vi "lab5_task3_2.vi"() -> ()   [LabVIEW 2021]
uses:
  <vilib>/express/express analysis/Spectral/Block/exnSpectralBlock spectral measurements PSD poly.vi
  <vilib>/express/express analysis/Spectral/Block/exnSpectralBlock spectral measurements PSD DDT.vi
  <vilib>/express/express analysis/Spectral/XNode/ExpressSpectralMeasurementsBlockNode.xnode
  <vilib>/Analysis/NI_AALPro.lvlib
panel:
  out "mass(g)":dbl
  out "number samples":dbl
  in  "Duration(s)":dbl=10000.0
  in  "Sampling rate(hz)":dbl=10000.0
  in  "stop":bool
  out "Intensity Chart":dbl[][](graph)
  out "Power spectral density":dynamicdata(graph)
  in  "# bins":i32
  out "Histogram Graph":T1(graph)
  out "rms":dbl
  out "peak to peak":dbl
  out "mean":dbl
  out "data":dynamicdata(graph)
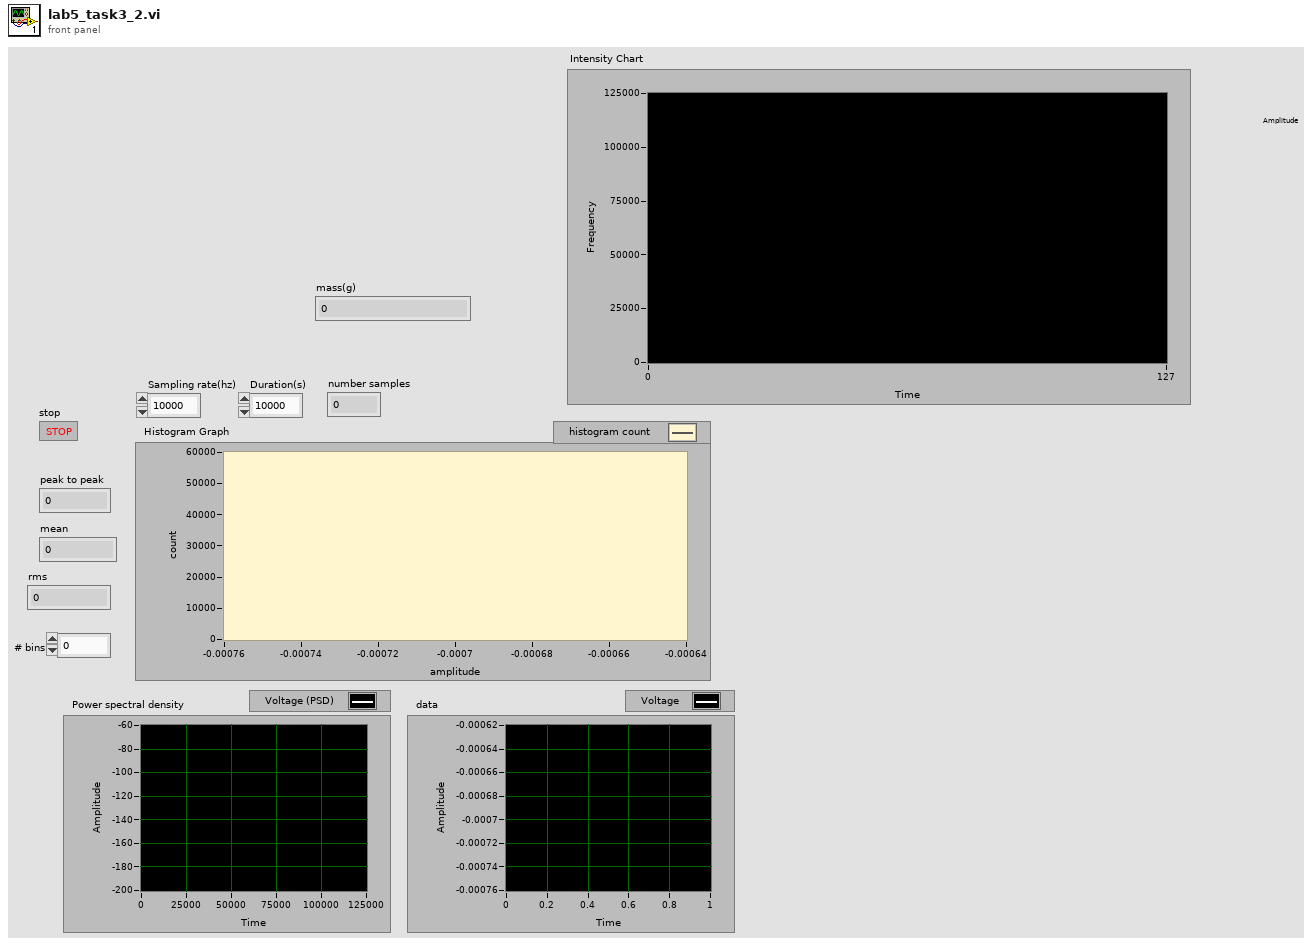
[diagram p1: front panel]
types:
  T1 = cluster{"X Values":dbl[], "Histogram: h(x)":i32[]}
  T2 = cluster{"averaging mode":u16, "weighting mode":u16, "number of averages":u32}
  T3 = cluster{"dB On (F)":bool, "unwrap phase (F)":bool, "convert to degree (F)":bool}
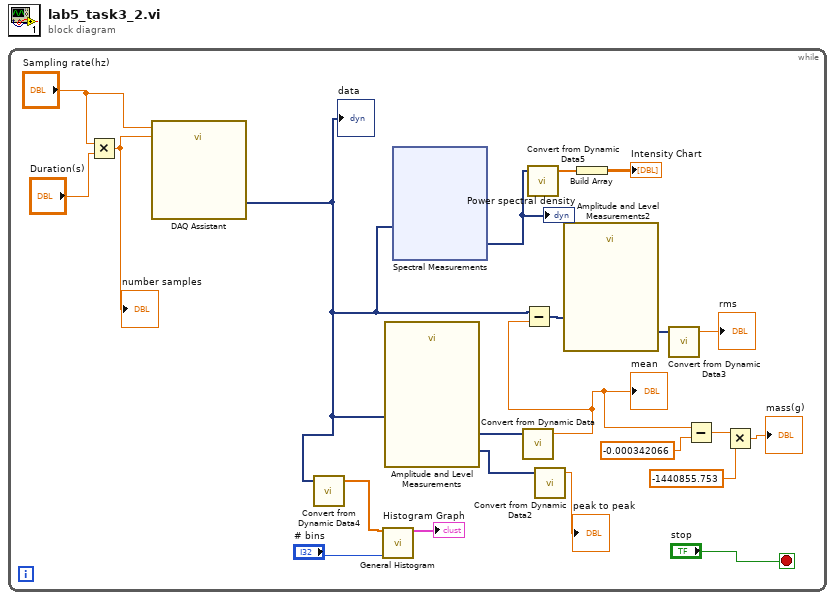
[diagram p0: block diagram]
diagram:
  n1 = while {
    stop <- "stop" stop-if-true
    n2 = Multiply(x="Sampling rate(hz)", y="Duration(s)") -> (x*y=w6:dbl)
    "number samples" <- w6
    n3 = call "DAQ Assistant"("rate"="Sampling rate(hz)", "number of samples"=w6) -> ("data"=w13:dynamicdata)  [unwired: 15 in, 2 out]
    "data" <- w13
    n4 = call "Convert from Dynamic Data4"("Dynamic Data Type"=w13) -> ("Array"=w14:dbl[])  [unwired: 3 in]
    n5 = call <vilib>:"General Histogram.vi"("X"=w14, "# bins"="# bins") -> ("Histogram Graph"=→"Histogram Graph":T1)  [unwired: 9 in, 4 out]
    n6 = call "Amplitude and Level Measurements"("Signals"=w13) -> ("Mean (DC)"=w22:dynamicdata, "Peak to Peak"=w21:dynamicdata)  [unwired: 12 in, 1 out]
    n7 = xnode "Spectral Measurements"("Signals"=w13) -> ("PSD"=w12:dynamicdata)  [unwired: 1 in, 1 out]
    "Power spectral density" <- w12
    n8 = call "Convert from Dynamic Data"("Dynamic Data Type"=w22) -> ("Scalar"=w5:dbl)  [unwired: 3 in]
    "mean" <- w5
    n9 = Subtract(x=w13, y=w5) -> (x-y=w19:dynamicdata)
    n10 = call "Convert from Dynamic Data5"("Dynamic Data Type"=w12) -> ("Array"=w11:dbl[])  [unwired: 3 in]
    n11 = call "Convert from Dynamic Data2"("Dynamic Data Type"=w21) -> ("Scalar"=→"peak to peak":dbl)  [unwired: 3 in]
    n12 = call "Amplitude and Level Measurements2"("Signals"=w19) -> ("RMS"=w18:dynamicdata)  [unwired: 13 in, 1 out]
    n13 = Build Array(w11) -> (→"Intensity Chart":dbl[][])
    n14 = call "Convert from Dynamic Data3"("Dynamic Data Type"=w18) -> ("Scalar"=→"rms":dbl)  [unwired: 3 in]
    n15 = Subtract(x=w5, y=-0.000342066) -> (x-y=w3:dbl)
    n16 = Multiply(x=w3, y=-1440855.753) -> (x*y=→"mass(g)":dbl)
  }
